vi "CopyROIOrigin.vi"(6 "Root":path, 8 "error in (no error)":errorcluster, 9 "ROI List":i32[](array[numeric]), 11 "Numbers":i32) -> (0 "error out":errorcluster)   [LabVIEW 2019]
uses:
  Controls/ROI_List_Action.ctl
  Analysis/Controls/Parttern Match/Analysis_PatternMatch_Parameter.ctl
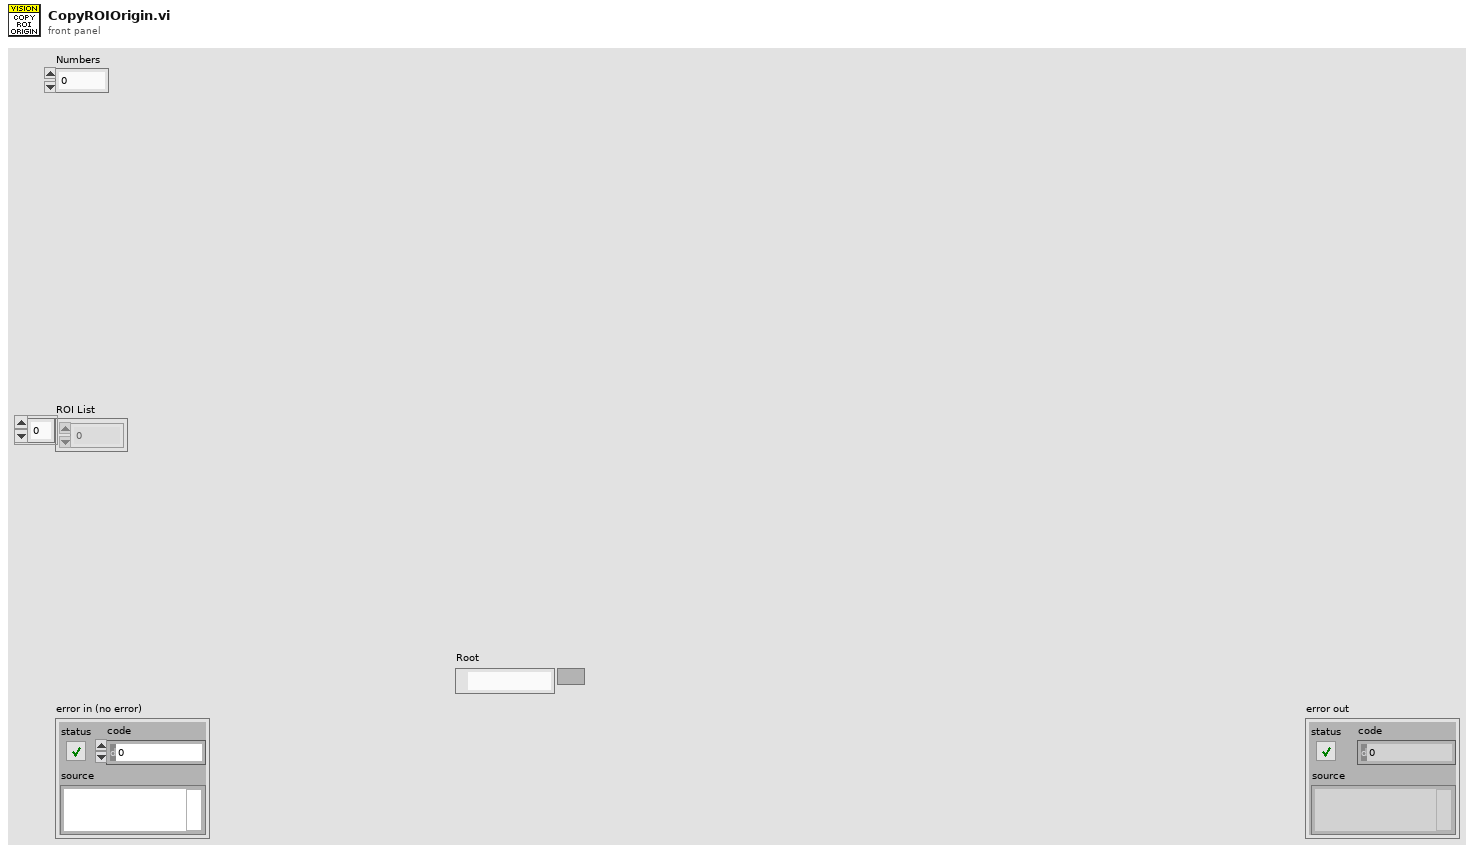
[diagram p1: front panel]
types:
  T1 = typedef "ROI_List_Action.ctl" = enum16{"Init", "Add ROI", "Delete ROI", "Get All ROI", "Get Specific ROI", "Set Analysis Setting", "Set Process Setting", "Replace All Entries", "ROIEntryBackup", "ROIEntryBackupClear", "ROIEntryReturn"}
  T2 = typedef "Vision_DataEntry.ctl" = cluster{"vROIName":string, "vROIContour":cluster{"Contour Type":u32, "ROI Type":u32, "Points":i32[]}, "ProcessSetting":T3[], "Analysis_Setting":T5}
  T3 = typedef "Process_Setting.ctl" = cluster{"Enum_PreProcess":T4, "Parameter":string}
  T4 = typedef "VisionProcessName.ctl" = enum16{"*CamParameter*", "CamAttributes", "*Preprocess*", "CG_Brightness", "C_Plane Extraction", "C_Threshold", "G_Lookup Table", "G_Threshold"}
  T5 = typedef "Analysis_Setting.ctl" = cluster{"PreProcess":T6, "Parameter":string}
  T6 = typedef "VisionProcessName.ctl" = enum16{"*CamParameter*", "CamAttributes", "*Preprocess*", "CG_Brightness", "C_Plane Extraction", "C_Threshold", "G_Lookup Table", "G_Threshold", "B_Image Inversion", "*Algorithm*", "CG_Histogram", "C_Color Matching", "C_Color Pattern Matching", "G_PatternMatch", "CG_Find Straight Edge", "CG_Adv. Find Straight Edge", "CG_Find Circular Edge", "G_Max Clamp", "G_Clamp (Rake)", "G_Pattern Matching"}
  T7 = cluster{"Contour Type":u32, "ROI Type":u32, "Points":i32[]}
  T8 = typedef "Analysis_PatternMatch_Parameter.ctl" = cluster{"Algorithm":i32, "Match Parameters":cluster{"Number of Matches Requested":i32, "Minimum Match Score":sgl, "Angle Ranges":cluster{"Start Angle":sgl, "End Angle":sgl}[]}, "ROI Descriptor":T9, "Advanced Options":cluster{"Item":u16, "Value":dbl}[], "Template path":string, "XOffset":i32, "YOffset":i32}
  T9 = typedef "ROI Descriptor" = cluster{"Global Rectangle":i32[], "Contours":cluster{"ID":enum32{"External", "Internal"}, "Type":u32, "Coordinates":i32[]}[]}
  T10 = typedef "Vision_DataEntry.ctl" = cluster{"vROIName":string, "vROIContour":cluster{"Contour Type":u32, "ROI Type":u32, "Points":i32[]}, "ProcessSetting":T3[], "Analysis_Setting":T11}
  T11 = typedef "Analysis_Setting.ctl" = cluster{"PreProcess":T12, "Parameter":string}
  T12 = typedef "V_Analysis_Type.ctl" = enum16{"None", "C_Color Pattern Matching", "G_PatternMatching", "G_ShapeDectect", "G_GeometricMatch", "B_Area Check"}
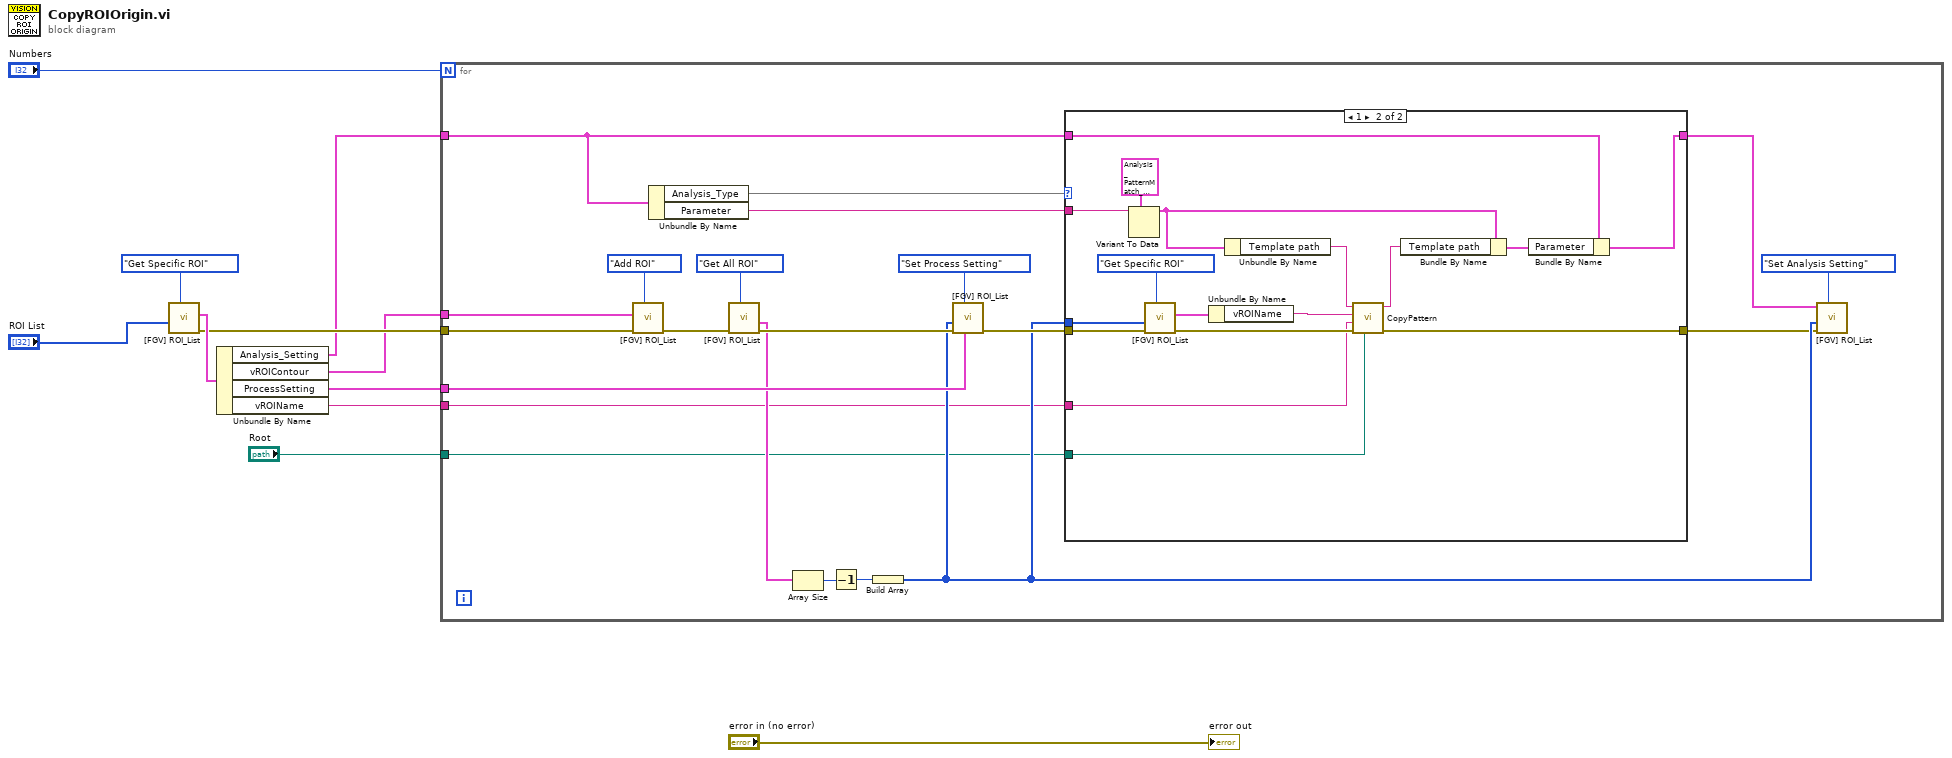
[diagram p0: block diagram]
diagram:
  n1 = call "[FGV] ROI_List.vi"("Action"=ROI_List_Action."Get Specific ROI", "ROIs_Index"="ROI List") -> ("error out"=w8:errorcluster, "ROI Entry"=w10:T2)  [unwired: 7 in, 1 out]
  n2 = Unbundle By Name(w10) -> ("Analysis_Setting"=w5:T5, "vROIContour"=w6:T7, "ProcessSetting"=w4:T3[], "vROIName"=w3:string)
  n3 = for {
    N: "Numbers" -> [_]
    tunnel: w4 -> [w30]
    tunnel: w8 -> [w28]
    tunnel: w6 -> [w27]
    tunnel: w5 -> [w15]
    tunnel: w3 -> [w13]
    tunnel: "Root" -> [w12]
    n4 = call "[FGV] ROI_List.vi"("Action"=ROI_List_Action."Add ROI", "error in (no error)"=w28, "ROI_To_Add"=w27) -> ("error out"=w25:errorcluster)  [unwired: 6 in, 2 out]
    n5 = Unbundle By Name(w15) -> ("Analysis_Type"=w19, "Parameter"=w21:string)
    n6 = call "[FGV] ROI_List.vi"("Action"=ROI_List_Action."Get All ROI", "error in (no error)"=w25) -> ("error out"=w24:errorcluster, "All ROI"=w23:T10[])  [unwired: 7 in, 1 out]
    n7 = Array Size(array=w23) -> (size(s)=w22:i32)
    n8 = Decrement(x=w22) -> (x-1=w20:i32)
    n9 = Build Array(w20) -> (w17:i32[])
    n10 = call "[FGV] ROI_List.vi"("ProcessSetting"=w30, "Action"=ROI_List_Action."Set Process Setting", "error in (no error)"=w24, "ROIs_Index"=w17) -> ("error out"=w18:errorcluster)  [unwired: 5 in, 2 out]
    n11 = case shown="1" w19 {
      tunnel: w21 -> [_ w50]
      tunnel: w18 -> [w33 w47]
      tunnel: w17 -> [_ w46]
      tunnel: [w33 w35] -> w16
      tunnel: w15 -> [w34 w44]
      tunnel: [w34 w42] -> w14
      tunnel: w13 -> [_ w37]
      tunnel: w12 -> [_ w36]
      frame Default {
      }
      frame 1 {
        n12 = Variant To Data(type=T8 {"Algorithm"=2, "Match Parameters"={"Number of Matches Requested"=1, "Minimum Match Score"=750.0, "Angle Ranges"=[]}, "ROI Descriptor"={"Global Rectangle"=[], "Contours"=[]}, "Advanced Options"=[{"Item"=1, "Value"=1.0}, {"Item"=103, "Value"=1.0}], "Template path"="", "XOffset"=0, "YOffset"=0} ("PatternMatchParameter"), Variant=w50) -> (data=w49:T8)  [unwired: 1 in, 1 out]
        n13 = call "[FGV] ROI_List.vi"("Action"=ROI_List_Action."Get Specific ROI", "error in (no error)"=w47, "ROIs_Index"=w46) -> ("error out"=w41:errorcluster, "ROI Entry"=w45:T2)  [unwired: 6 in, 1 out]
        n14 = Unbundle By Name(w45) -> ("vROIName"=w38:string)
        n15 = Unbundle By Name(w49) -> ("Template path"=w40:string)
        n16 = call "CopyPattern.vi"("Root"=w36, "error in (no error)"=w41, "SourceName"=w37, "CopyName"=w38, "SourcePatternPath"=w40) -> ("error out"=w35:errorcluster, "CopyPatternPath"=w39:string)  [unwired: 5 in]
        n17 = Bundle By Name(cluster=w49, "Template path"=w39) -> (w43:T8)
        n18 = Bundle By Name(cluster=w44, "Parameter"=w43) -> (w42:T5)
      }
    }
    n19 = call "[FGV] ROI_List.vi"("Action"=ROI_List_Action."Set Analysis Setting", "error in (no error)"=w16, "ROIs_Index"=w17, "Analysis_Setting"=w14) -> ()  [unwired: 5 in, 3 out]
  }
  "error out" <- "error in (no error)"
